vi "Pruebaciclo2.vi"() -> ()   [LabVIEW 2013]
panel:
  out "Mucha Calor":bool
  out "Contador":dbl
  out "Temperatura Promedio":dbl
  out "Temperatura Mayor":dbl
  out "Thermometer":i32(slide) scale=0.0..100.0
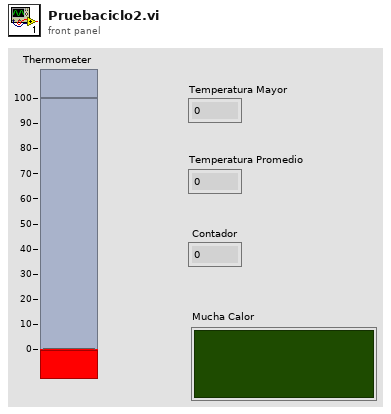
[diagram p1: front panel]
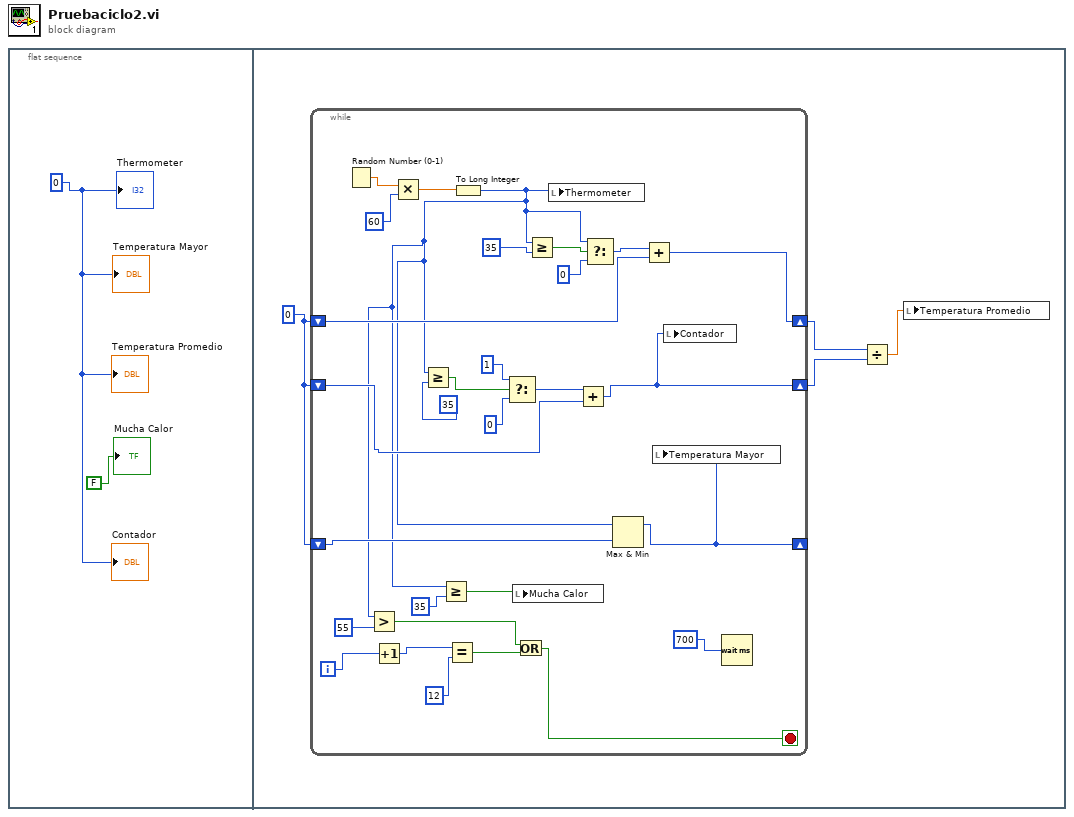
[diagram p0: block diagram]
diagram:
  n1 = flat-sequence {
    frame #0 {
      w2 = 0
      "Thermometer" <- w2
      "Temperatura Promedio" <- w2
      "Contador" <- w2
      "Temperatura Mayor" <- w2
      "Mucha Calor" <- FALSE
    }
    frame #1 {
      w3 = 0
      n2 = while {
        shift-right: [w27] -> w5
        shift-left: w3 -> [w29]
        shift-right: [w21] -> w4
        shift-left: w3 -> [w12]
        shift-right: [w19] -> _
        shift-left: w3 -> [w20]
        i -> [w15]
        stop <- w8 stop-if-true
        n3 = Random Number (0-1)() -> (number: 0 to 1=w35:dbl)
        n4 = Increment(x=w15) -> (x+1=w13:i32)
        n5 = Multiply(x=w35, y=60) -> (x*y=w34:dbl)
        n6 = Equal?(x=w13, y=12) -> (x = y?=w9:bool)
        n7 = To Long Integer(number=w34) -> (32bit integer=w7:i32)
        n8 = Greater?(x=w7, y=55) -> (0:w10:bool)
        n9 = Greater Or Equal?(x=w7, y=35) -> (x >= y?=w24:bool)
        n10 = Greater Or Equal?(x=w7, y=35) -> (x >= y?=w18:bool)
        n11 = Select(t=1, s=w24, f=0) -> (s? t:f=w22:i32)
        n12 = local write "Mucha Calor"(w18) -> ()
        n13 = Or(x=w10, y=w9) -> (x .or. y?=w8:bool)
        n14 = Greater Or Equal?(x=w7, y=35) -> (x >= y?=w30:bool)
        n15 = local write "Thermometer"(w7) -> ()
        n16 = Add(x=w22, y=w12) -> (x+y=w21:i32)
        n17 = Select(t=w7, s=w30, f=0) -> (s? t:f=w28:i32)
        n18 = Max & Min(x=w7, y=w20) -> (max(x,y)=w19:i32)  [unwired: 1 out]
        n19 = Add(x=w28, y=w29) -> (x+y=w27:i32)
        n20 = local write "Temperatura Mayor"(w19) -> ()
        n21 = local write "Contador"(w21) -> ()
        n22 = Wait (ms)(milliseconds to wait=700) -> ()  [unwired: 1 out]
      }
      n23 = Divide(x=w5, y=w4) -> (x/y=w6:dbl)
      n24 = local write "Temperatura Promedio"(w6) -> ()
    }
  }
